vi "SetActiveMeasFunc.vi"(8 "error in (no error)":errorcluster caption="entrée d'erreur (pas d'erreur)", 9 "ItemIndex":i32, 10 "ListRef":refnum<vi>, 11 "Experiment en entrée":refnum<class "Experiment.lvclass"> caption="DNL_LabVIEW Object in") -> (0 "error out":errorcluster caption="sortie d'erreur", 3 "Experiment en sortie":refnum<class "Experiment.lvclass"> caption="DNL_LabVIEW Object out")   [LabVIEW 2019, in "Experiment.lvclass"]
uses:
  Experiment.lvclass
  Experiment.lvclass/Experiment.ctl
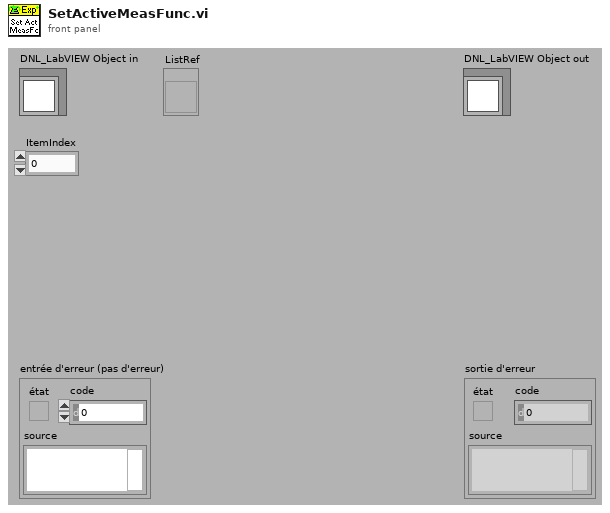
[diagram p1: front panel]
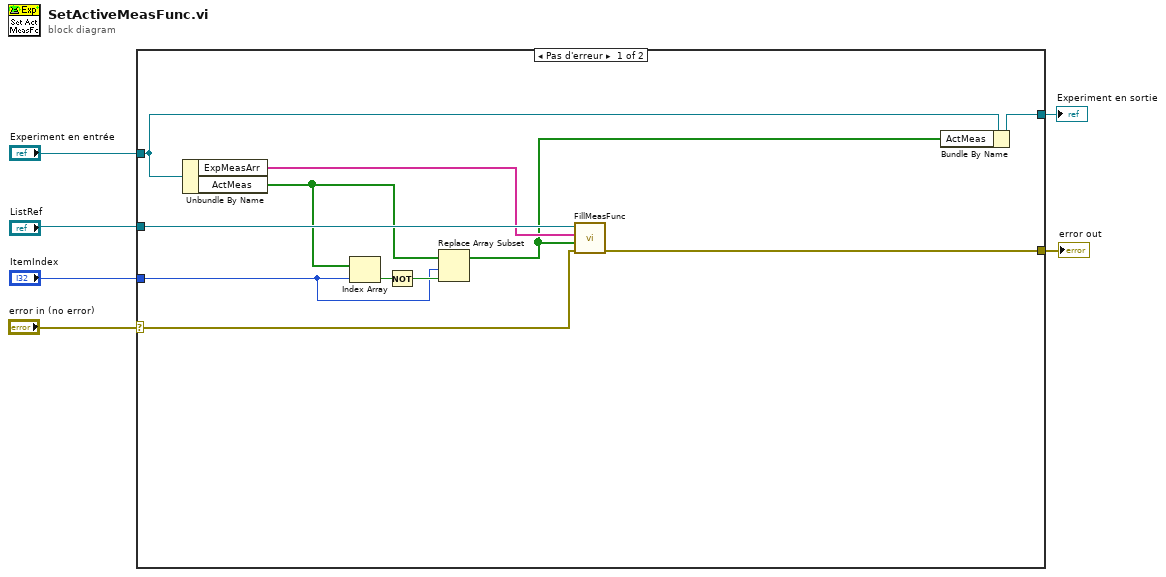
[diagram p0: block diagram]
diagram:
  n1 = case shown="Pas d'erreur" "error in (no error)" {
    selector: "error in (no error)" -> [w16 w19]
    tunnel: [w7 w19] -> w5
    tunnel: [w12 w18] -> w3
    tunnel: "Experiment en entrée" -> [w17 w18]
    tunnel: "ListRef" -> [w13 _]
    tunnel: "ItemIndex" -> [w11 _]
    frame No Error {
      n2 = Unbundle By Name(w17) -> ("ExpMeasArr"=w9:string[], "ActMeas"=w10:bool[])
      n3 = Index Array(array=w10, index=w11) -> (element=w15:bool)
      n4 = Not(x=w15) -> (.not. x?=w14:bool)
      n5 = Replace Array Subset(array=w10, new element=w14, index=w11) -> (w8:bool[])
      n6 = call "FillMeasFunc.vi"("ErrorIn(No Error)"=w16, "ActMeas"=w8, "MeasFunc"=w9, "ListRef"=w13) -> ("sortie d'erreur"=w7:errorcluster)  [unwired: 6 in, 1 out]
      n7 = Bundle By Name(cluster=w17, "ActMeas"=w8) -> (w12:refnum<class "Experiment.lvclass">)
    }
    frame Error {
    }
  }
  "error out" <- w5
  "Experiment en sortie" <- w3
